vi "Write Yields.vi"(5 "General.Sequence Path":path, 6 "Station":i32, 7 "Socket":i32, 8 "error in (no error)":errorcluster, 10 "Failed":i32, 11 "Totals":i32) -> (0 "error out":errorcluster)   [LabVIEW 2025, in "Test Unit.lvlib"]
uses:
  Test Unit.lvlib
  <vilib>/Utility/config.llb/Write Key (I32).vi
  Full User Interface/Full User Interface.lvlib
  <vilib>/Utility/config.llb/NI_LVConfig.lvlib
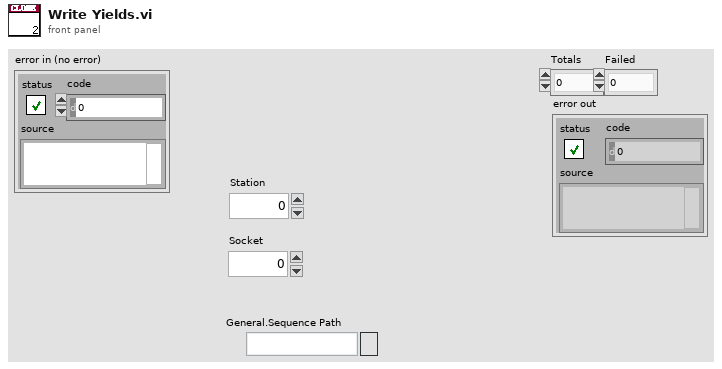
[diagram p1: front panel]
types:
  T1 = typedef "NI_LVConfig.lvlib/Config Data RefNum.ctl" = refnum<k1>
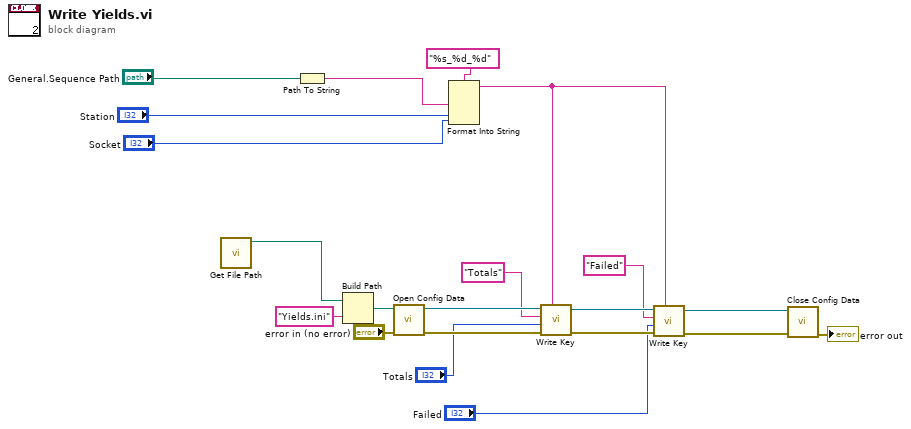
[diagram p0: block diagram]
diagram:
  n1 = call "Get File Path.vi"() -> ("Application Directory"=w21:path)  [unwired: 11 in]
  n2 = Path To String(path="General.Sequence Path") -> (string=w11:string)
  n3 = Build Path(base path=w21, name or relative path="Yields.ini") -> (appended path=w19:path)
  n4 = call <vilib>:"Open Config Data.vi"("error in (no error)"="error in (no error)", "configuration file path"=w19) -> ("error out"=w14:errorcluster, "refnum"=w18:T1)  [unwired: 7 in, 1 out]
  n5 = Format Into String(format string="%s_%d_%d", w11, "Station", "Socket") -> (resulting string=w10:string)  [unwired: 2 in, 1 out]
  n6 = call-poly <vilib>:"Write Key.vi"("section"=w10, "error in (no error)"=w14, "value"="Totals", "key"="Totals", "refnum"=w18) -> ("error out"=w13:errorcluster, "refnum out"=w16:T1)  [unwired: 4 in, 1 out]
  n7 = call-poly <vilib>:"Write Key.vi"("section"=w10, "error in (no error)"=w13, "value"="Failed", "key"="Failed", "refnum"=w16) -> ("error out"=w7:errorcluster, "refnum out"=w8:T1)  [unwired: 4 in, 1 out]
  n8 = call <vilib>:"Close Config Data.vi"("error in (no error)"=w7, "refnum"=w8) -> ("error out"=→"error out":errorcluster)  [unwired: 8 in, 1 out]
